vi "Init.vi"(8 "error in":errorcluster, 11 "SEQ in":refnum<class "SEQ.lvclass">) -> (0 "error out":errorcluster, 3 "SEQ out":refnum<class "SEQ.lvclass">)   [LabVIEW 2015, in "Sequence Composition.lvlib" / "SEQ.lvclass"]
doc: "Grab a reference to a queue for the sequence steps and set the first call value to TRUE."
uses:
  SEQ.lvclass
  STEPS/STEP.lvclass
  SEQ.lvclass/SEQ.ctl
  STEPS/STEP.lvclass/STEP.ctl
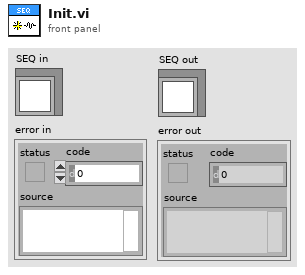
[diagram p1: front panel]
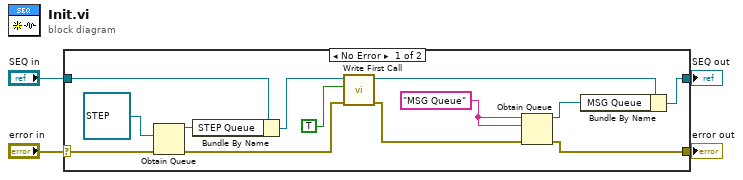
[diagram p0: block diagram]
diagram:
  n1 = case shown="No Error" "error in" {
    selector: "error in" -> [w16 w19]
    tunnel: [w5 w19] -> w3
    tunnel: [w7 w18] -> w1
    tunnel: "SEQ in" -> [w15 w18]
    frame No Error {
      w9 = "MSG Queue" ("name (unnamed)")
      n2 = Obtain Queue(element data type=refnum<class "STEP.lvclass"> refnum ("STEP.lvclass"), error in (no error)=w16) -> (queue out=w14:refnum<queue>, error out=w12:errorcluster)  [unwired: 3 in, 1 out]
      n3 = Bundle By Name(cluster=w15, "STEP Queue"=w14) -> (w13:refnum<class "SEQ.lvclass">)
      n4 = call "Write First Call.vi"("error in"=w12, "First Call?"=TRUE, "STEP in"=w13) -> ("error out"=w10:errorcluster, "STEP out"=w8:refnum<class "SEQ.lvclass">)  [unwired: 7 in]
      n5 = Obtain Queue(name (unnamed)=w9, element data type=w9, error in (no error)=w10) -> (queue out=w6:refnum<queue>, error out=w5:errorcluster)  [unwired: 2 in, 1 out]
      n6 = Bundle By Name(cluster=w8, "MSG Queue"=w6) -> (w7:refnum<class "SEQ.lvclass">)
    }
    frame Error {
    }
  }
  "error out" <- w3
  "SEQ out" <- w1
